vi "Plotter_TDMS.vi"() -> ()   [LabVIEW 2020]
uses:
  General-Controler/panel position.ctl
  Shared/MySQL/Preset Query Enum.ctl
  plotter setup cluster.ctl
  <vilib>/Utility/tcp.llb/UDP Multicast Read-Only Open.vi
  <userlib>/_OpenG.lib/file/file.llb/Convert File Extension (Path)__ogtk.vi
panel:
  in  "Stop button":bool
  in  "Tab Control 2":T1(tab)
  out "parameters to get":string[][](array[string])
  out "devices to get data from":string[](array[string])
  out "Mcast Data":string
  out "scans path":path
  out "TDMS file path":path
  out "Axis Name List":string[](array[string])
  out "All Devices Core Info":string[][](array[string])
  out "UDP Mcast Error":errorcluster
  out "plotter details":string[][](array[string])
  in  "Cluster":T2
  out "appargs":string[](array[string])
  in  "Tab Control":T3(tab)
  out "xy graph":cluster{dbl[], dbl[]}[](graph)
  out "Scan":string
  out "Scan in progress":bool
  out "xy graph bin":cluster{dbl[], dbl[]}[](graph)=[{[5.5, 15.5, 25.5, 35.5, 45.5, 55.5, 0.0], [0.1, 0.1, 0.15, 0.15, 0.2, 0.2, 0.0]}, {[5.5, 5.5, nan, 15.5, 15.5, nan, 25.5, 25.5, nan, 35.5, 35.5, nan, 45.5, 45.5, nan, 55.5, 55.5, nan, 0.0, 0.0, nan], [0.1, 0.1, nan, 0.1, 0.1, nan, 0.15, 0.15, nan, 0.15, 0.15, nan, 0.2, 0.2, nan, 0.2, 0.2, nan, 0.0, 0.0, nan]}, {[5.5, 15.5, 25.5, 35.5, 45.5, 55.5, 0.0], [5.5, 15.5, 25.5, 35.5, 45.5, 55.5, 0.0]}, {[5.5, 5.5, nan, 15.5, 15.5, nan, 25.5, 25.5, nan, 35.5, 35.5, nan, 45.5, 45.5, nan, 55.5, 55.5, nan, 0.0, 0.0, nan], [3.0, 8.0, nan, 13.0, 18.0, nan, 23.0, 28.0, nan, 33.0, 38.0, nan, 43.0, 48.0, nan, 53.0, 58.0, nan, 0.0, 0.0, nan]}]
  in  "Override":bool
  out "Experiment":u16(ring) items=["BaratronProject", "Bella", "ControlRoom", "DataLogging", "Developer", "HeaterTest", "Lanex Bella", "Plasma2", "Test"]
  out "Current State":string
  out "Mcast Path Data":string
  in  "file path":path
  in  "FilePath":bool
  in  "replot":bool
  in  "X Axis":u16(ring)=1
  in  "Y Axis 2":u16(ring)
  in  "Y Axis":u16(ring)
  in  "override":bool
  in  "replot 2":bool
  in  "y axis 2 override":string
  in  "y axis override":string
  in  "x axis override":string
  out "device data Spreadsheet format":string[][](array[string])
  in  "Left":i16=25
  in  "Top":i16=75
  in  "expt_Plotteridfor vi mode":string="46"
  out "Actual expt_plotter.id":string
  out "expt":string
  out "plotter#":string
  out "Screen\nPosition":cluster{"Left":i16, "Top":i16}
  out "x axis name":string
  out "ScanStart ExptName":string
  out "Y Axis Default name":string
  out "MC_IP":string
  out "Path used":path
  out "error out 2":errorcluster
  out "ScanStatus":string
  out "error out 5":errorcluster
  out "s start dat":string
  out "scan end mcast":string
  out "Y Axis Default name 2":string
  out "data":string[][](array[string])
  out "tdms data":string[][](array[string])
  # "17 Fake cam 1 to 5"
  # "15"
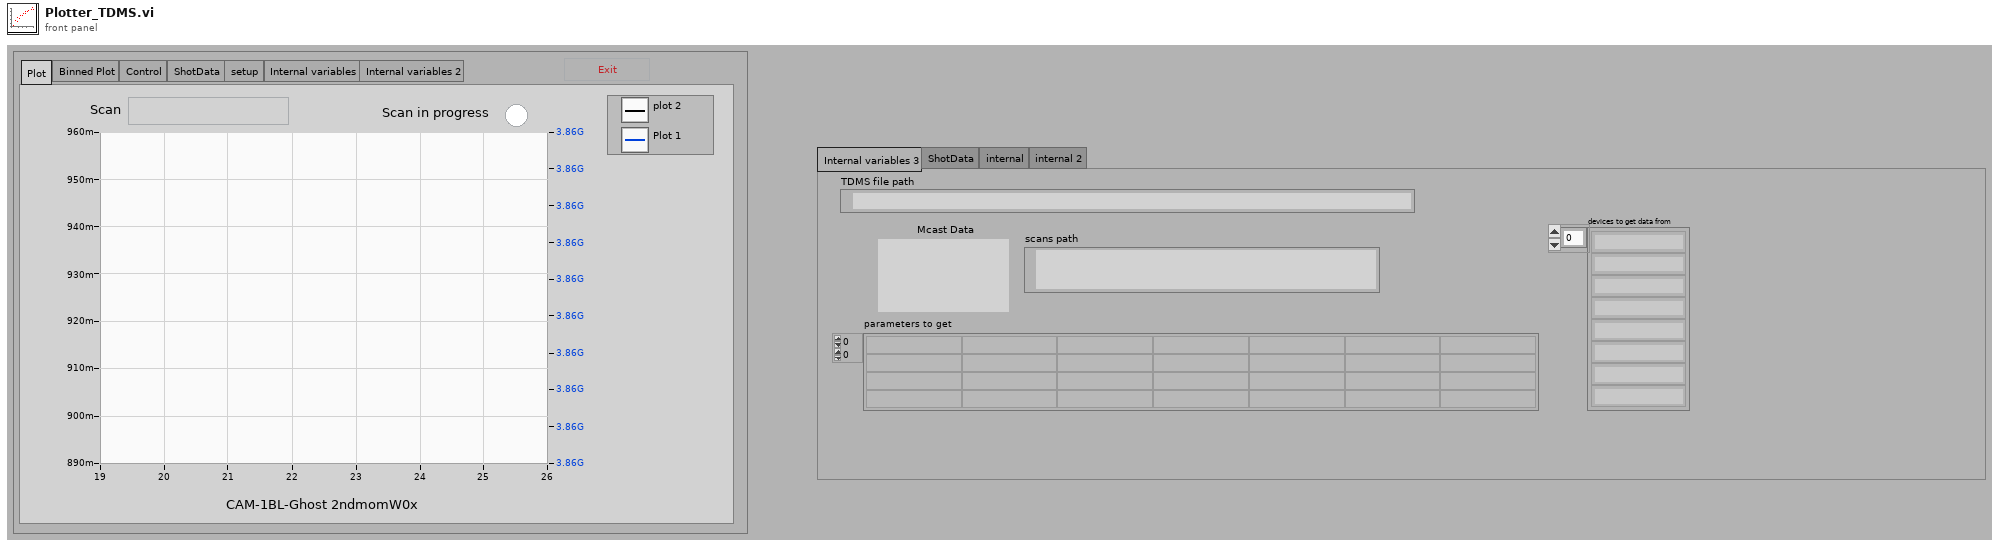
[diagram p1: front panel]
types:
  T1 = enum32{"Internal variables 3", "ShotData", "internal", "internal 2"}
  T2 = typedef "panel position.ctl" = cluster{"Left":i16, "Top":i16, "Width":u32, "Height":u32}
  T3 = enum32{"Plot", "Binned Plot", "Control", "ShotData", "setup", "Internal variables", "Internal variables 2"}
  T4 = typedef "Plotter FGV cluster control.ctl" = cluster{"Multicast Address":string, "Plotter Busy":bool, "Plotter Exit":bool, "Mcast Port":u16}
  T5 = enum32{"invalid app kind", "Development System", "Run Time System", "Student Edition", "Embedded LabVIEW", "Evaluation", "Custom"}
  T6 = enum32{"Invalid", "Standard", "Closed", "Hidden", "Minimized", "Maximized"}
  T7 = typedef "Preset Query Enum.ctl" = enum16{"Get Locations", "Get all IPs and MACs", "Get classes", "Get expt variables to set at scanstart for particular device", "Get expt devices and variables with start values", "Get expt devices and variables (with data to get)", "Get expt devices with data to get", "Get Expt devices and GUIs", "Get all devices basic properties", "Get Virtual Devices Core Info", "Get Expt names", "Get experiment basic properties", "Get experiment alarm variables", "Get MC Ports", "Get device network comm port", "Get devicetype lvclass path", "Get basic device properties", "Get Init Order", "Get all setable variables of a device", "Get device variable aliases", "Get force values of all settable variables", "Get all variables of a devicetype", "Get all variables of a device", "Get plotter details", "Get Saved Scans", "Get Scan Info", "GetGeneralGUIs", "Get expt for plotter", "Get plotter IDs from expt", "Get all devices", "Get all Virtual Devices", "Get all aliases", "Get variable and device info for Virtual Device", "GetItemLocatorIP", "Get IPs for GUIs", "Get DeviceType from Device", "GetLocalPortRange", "GetDevicePresetVariables", "Get Device Configuration", "GetAllPresetNames", "GetAllConfigurationNames", "GetPresetDeviceNames", "GetDeviceAliases", "GetDevicesOfClass"}
  T8 = typedef "plotter setup cluster.ctl" = cluster{"screenx":i16, "screeny":i16, "variable1":string, "variable2":string, "name":string}
  T9 = cluster{"Ring Refnum x":refnum<vi>, "Ring Refnum y":refnum<vi>, "Ring Refnum y 2":refnum<vi>, "XY Graph Refnum":refnum<vi>}
  T10 = cluster{"Core":cluster{"Current VI Reference":refnum<vi>, "Close Panel on Exit?":bool}, "All Devices Core Info":string[][], "Expt Config Files":string[], "Experiment name":string, "ScanData to receive":string[][], "Device Names for scan data":string[], "expt config file array":string[][], "Data titles from config array":string[], "TDMS file path":path, "Plotter setup cluster":T8, "plotter#":string, "bin complete":bool}
  T11 = typedef "LVRectTypeDef.ctl" = cluster{"Left":i16, "Top":i16, "Right":i16, "Bottom":i16}
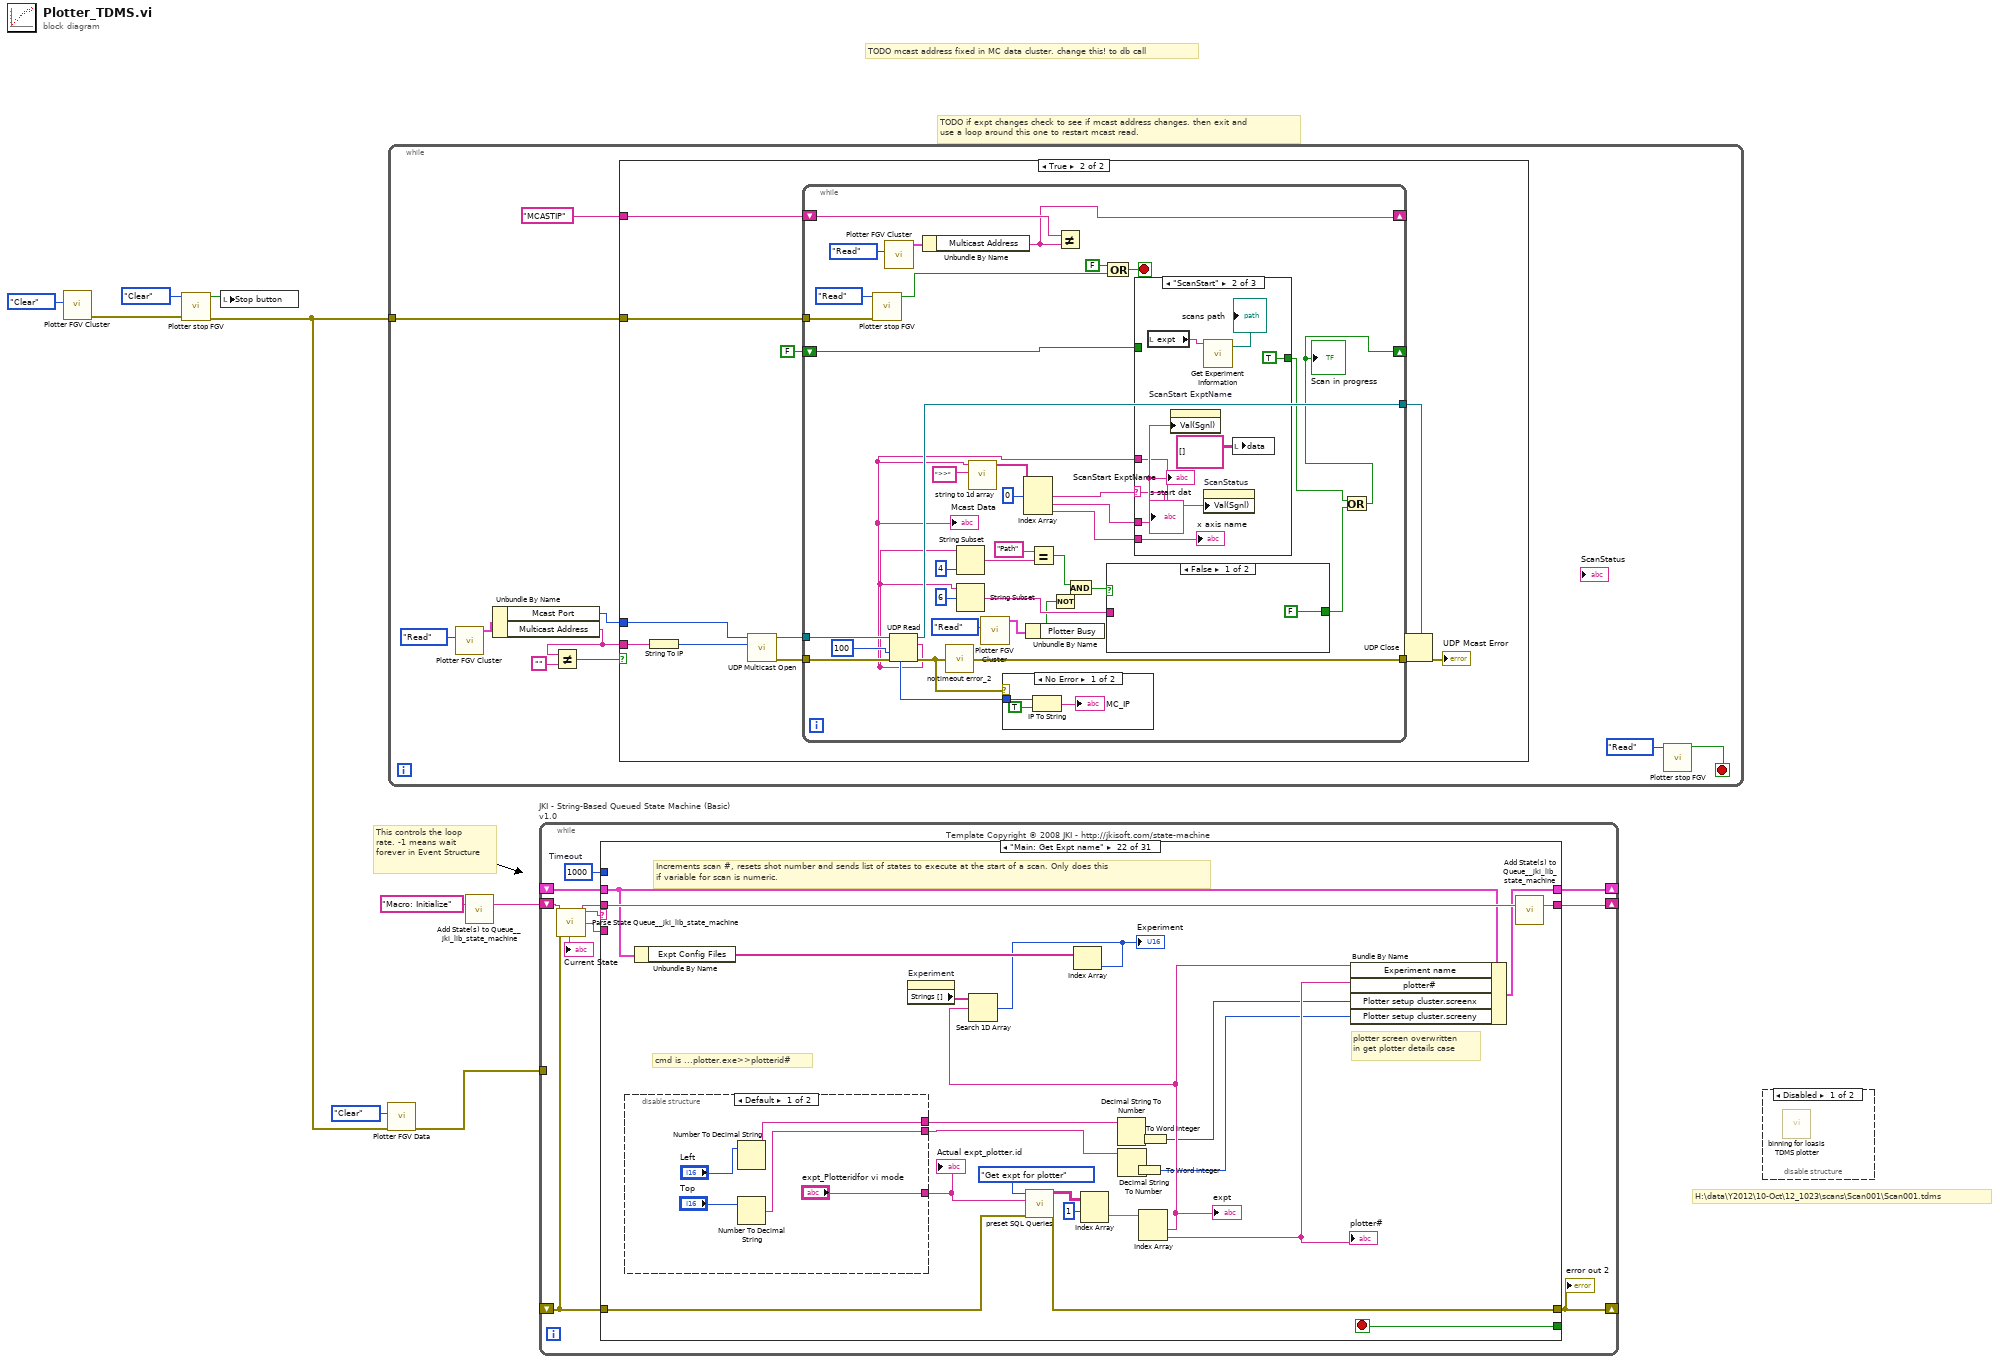
[diagram p0: block diagram]
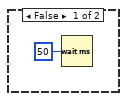
[diagram p3: hidden frame]
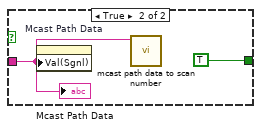
[diagram p5: hidden frame]
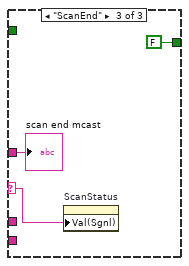
[diagram p7: hidden frame]
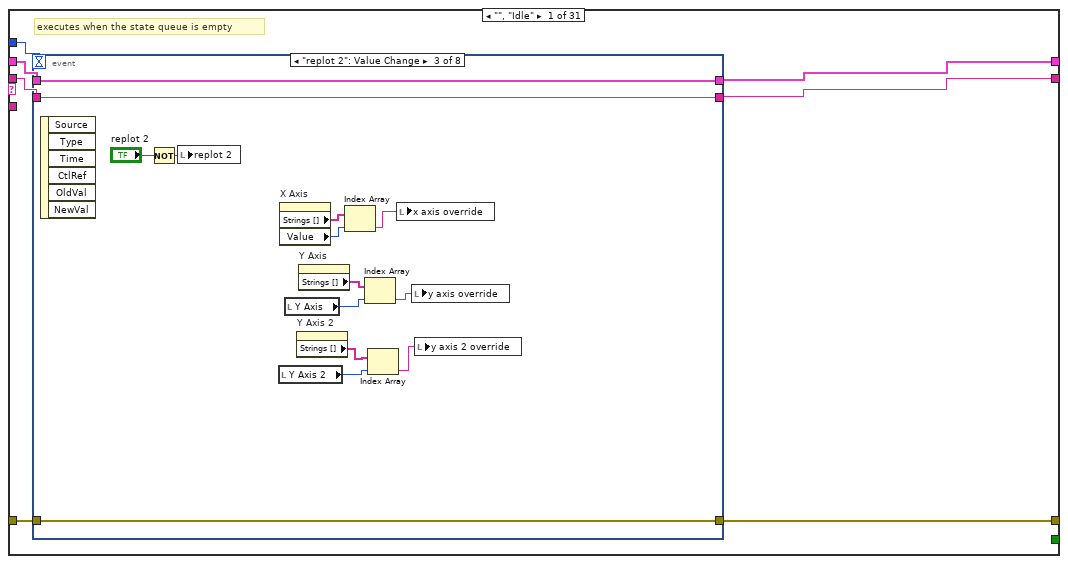
[diagram p8: hidden frame]
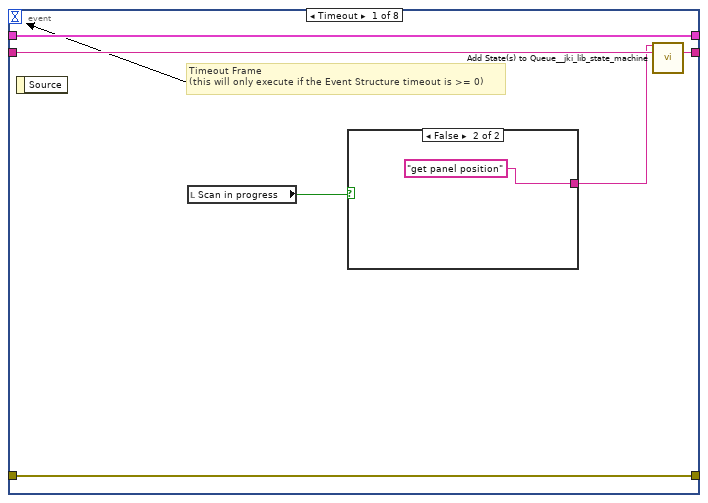
[diagram p9: hidden frame]
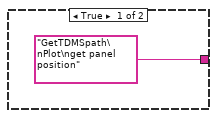
[diagram p10: hidden frame]
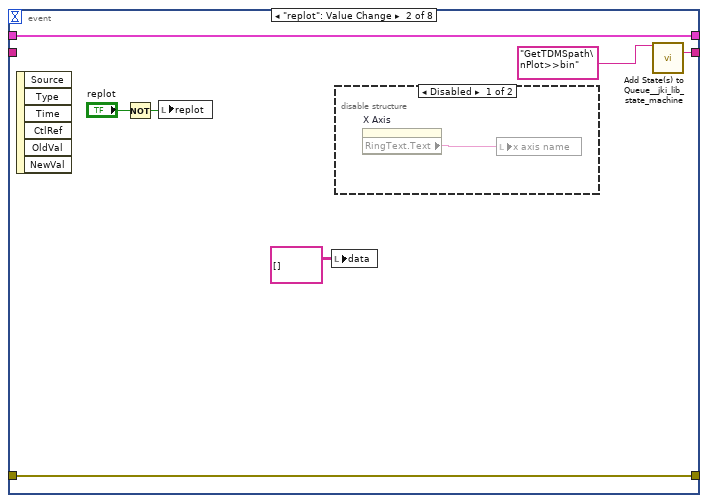
[diagram p11: hidden frame]
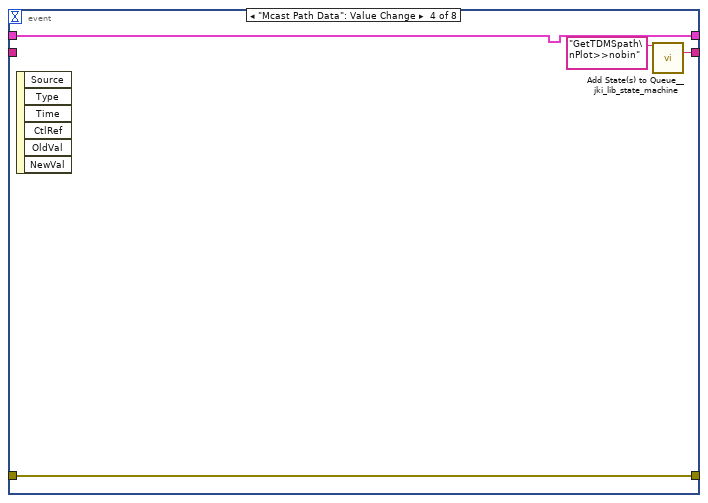
[diagram p13: hidden frame]
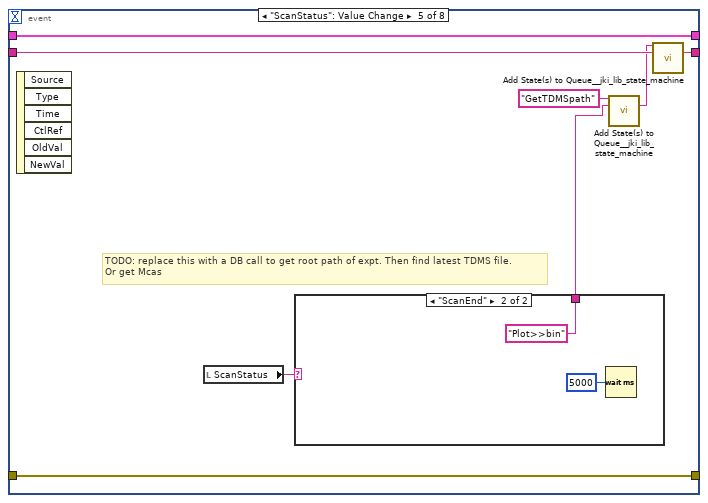
[diagram p14: hidden frame]
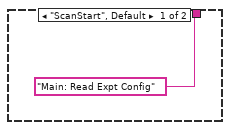
[diagram p15: hidden frame]
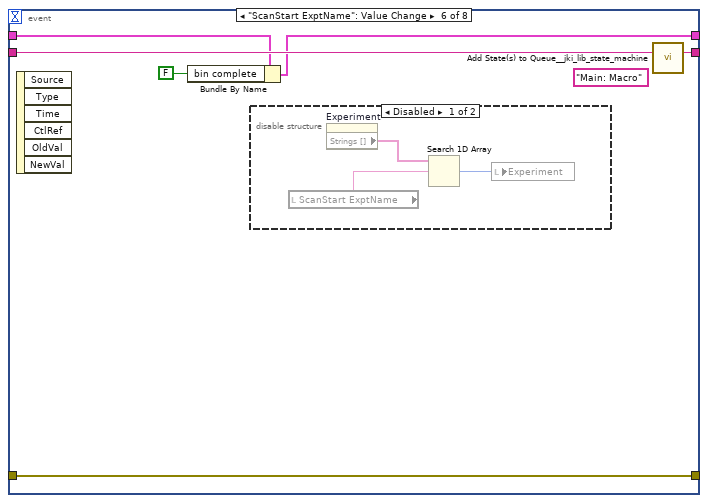
[diagram p16: hidden frame]
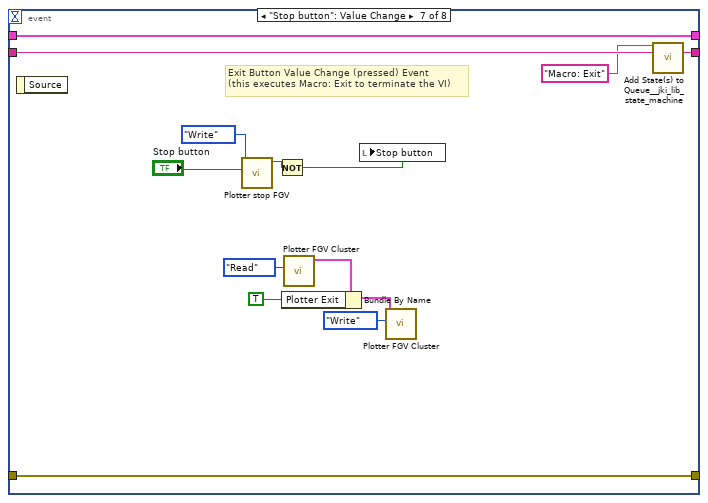
[diagram p18: hidden frame]
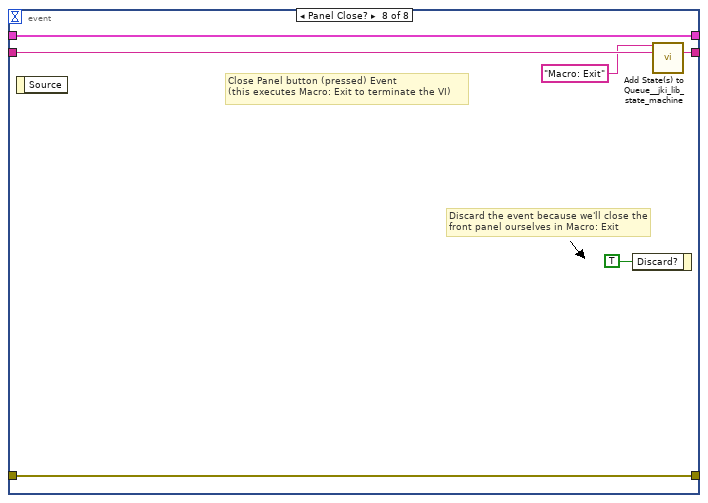
[diagram p19: hidden frame]
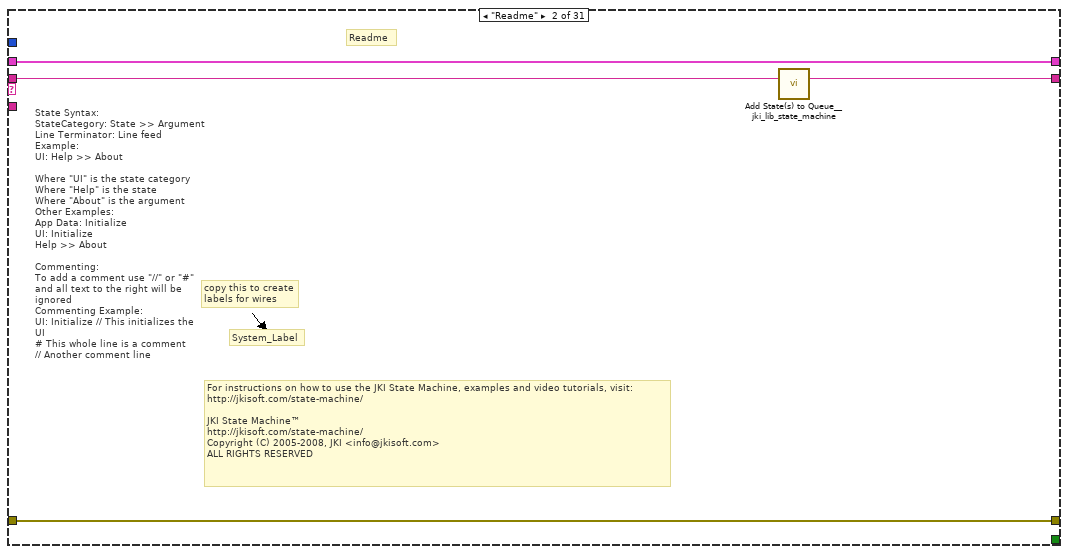
[diagram p20: hidden frame]
diagram:
  # "H:\\data\\Y2012\\10-Oct\\12_1023\\scans\\Scan001\\Scan001.tdms"
  # "TODO mcast address fixed in MC data cluster. change this! to db call"
  # "TODO if expt changes check to see if mcast address changes. then exit and\nuse a loop around this one to restart mcast read."
  # "This controls the loop rate. -1 means wait forever in Event Structure"
  n1 = call "Plotter FGV Cluster.vi"("Function"=enum16{"Read", "Write", "Clear"}."Clear") -> ("error out"=w5:errorcluster)  [unwired: 9 in, 1 out]
  n2 = call "Plotter stop FGV.vi"("error in"=w5, "Function"=enum16{"Read", "Write", "Clear"}."Clear") -> ("error out"=w2:errorcluster, "Stop out"=w4:bool)  [unwired: 8 in]
  n3 = local write "Stop button"(w4) -> ()
  n4 = call "Plotter FGV Data.vi"("error in"=w2, "Function"=enum16{"Read", "Write", "Clear"}."Clear") -> ("error out"=w1:errorcluster)  [unwired: 8 in, 1 out]
  n5 = while {
    tunnel: w2 -> [w13]
    stop <- w17 stop-if-true
    n6 = call "Plotter FGV Cluster.vi"("Function"=enum16{"Read", "Write", "Clear"}."Read") -> ("Cluster out"=w14:T4)  [unwired: 9 in, 1 out]
    n7 = Unbundle By Name(w14) -> ("Mcast Port"=w10:u16, "Multicast Address"=w12:string)
    n8 = Not Equal?(x=w12, y="") -> (x != y?=w16:bool)
    n9 = case shown="True" w16 {
      tunnel: "MCASTIP" ("Multicast Address") -> [_ w25]
      tunnel: w12 -> [_ w24]
      tunnel: w13 -> [_ w23]
      tunnel: w10 -> [_ w22]
      frame False {
        n10 = Wait (ms)(milliseconds to wait=u32 50) -> ()  [unwired: 1 out]
      }
      frame True {
        n11 = String To IP(1:w24) -> (0:w31:u32)
        n12 = call-poly <vilib>:"UDP Multicast Open.vi"("multicast addr"=w31, "port"=w22) -> ("error out"=w26:errorcluster, "connection ID"=w30:refnum<k16>)  [unwired: 7 in, 1 out]
        n13 = while {
          tunnel: w30 -> [w68]
          tunnel: [w67] -> w29
          tunnel: [w66] -> w28
          tunnel: w26 -> [w62]
          tunnel: w23 -> [w60]
          shift-right: [w38] -> _
          shift-left: w25 -> [w49]
          shift-right: [w34] -> _
          shift-left: FALSE -> [w33]
          stop <- w50 stop-if-true
          n14 = call "Plotter stop FGV.vi"("error in"=w60, "Function"=enum16{"Read", "Write", "Clear"}."Read") -> ("Stop out"=w51:bool)  [unwired: 8 in, 1 out]
          n15 = call "Plotter FGV Cluster.vi"("Function"=enum16{"Read", "Write", "Clear"}."Read") -> ("Cluster out"=w48:T4)  [unwired: 9 in, 1 out]
          n16 = UDP Read(connection ID=w68, timeout ms (25000)=100, 8:w62) -> (data out=w37:string, error out=w39:errorcluster, 3:w67:refnum<k16>, 6:w40:u32)  [unwired: 2 out]
          "Mcast Data" <- w37
          n17 = Unbundle By Name(w48) -> ("Multicast Address"=w38:string)
          n18 = call "no timeout error_2.vi"("error in (no error)"=w39) -> ("error out"=w66:errorcluster)
          n19 = String Subset(string=w37, length (rest)=4 ("length (rest)")) -> (substring=w57:string)  [unwired: 1 in]
          n20 = String Subset(string=w37, offset (0)=6) -> (substring=w55:string)  [unwired: 1 in]
          n21 = call "string to 1d array.vi"("delimiter (Tab)"=">>", "string"=w37) -> ("Array of Strings"=w64:string[])  [unwired: 9 in]
          n22 = call "Plotter FGV Cluster.vi"("Function"=enum16{"Read", "Write", "Clear"}."Read") -> ("Cluster out"=w43:T4)  [unwired: 9 in, 1 out]
          n23 = case shown="No Error" w39 {
            tunnel: w40 -> [w72 _]
            frame No Error {
              n24 = IP To String(1:TRUE ("dot notation? (F)"), 2:w72) -> (0:→"MC_IP":string)
            }
            frame Error {
            }
          }
          n25 = Index Array(array=w64, index #1=0 ("index")) -> (element #1=w46:string, element #2=w52:string, element #3=w53:string)  [unwired: 2 in]
          n26 = Unbundle By Name(w43) -> ("Plotter Busy"=w42:bool)
          n27 = Equal?(x="Path" ("y"), y=w57) -> (x = y?=w54:bool)
          n28 = Not(x=w42) -> (.not. x?=w41:bool)
          n29 = Not Equal?(x=w49, y=w38) -> ()  [unwired: 1 out]
          n30 = And(x=w54, y=w41) -> (x .and. y?=w45:bool)
          n31 = case shown="False" w45 {
            tunnel: w55 -> [_ w75]
            tunnel: [FALSE ("Scan in progress") TRUE ("Scan in progress")] -> w35
            frame False {
            }
            frame True {
              n32 = property on="Mcast Path Data" class="Str"("Val(Sgnl)"=w75) -> ()  [unwired: 2 in, 2 out]
              n33 = call "mcast path data to scan number.vi"("mcast path data"=w75) -> ()  [unwired: 10 in, 1 out]
              "Mcast Path Data" <- w75
            }
          }
          n34 = Compound Arithmetic op=OR(FALSE ("value"), w51) -> (w50:bool)
          n35 = case shown="\"ScanStart\"" w46 {
            selector: w46 -> [_ w82 w87]
            tunnel: w53 -> [_ w84 _]
            tunnel: w52 -> [_ w83 _]
            tunnel: w37 -> [_ w81 w86]
            tunnel: [w76 TRUE ("Scan in progress") FALSE ("Scan in progress")] -> w36
            tunnel: w33 -> [w76 _ _]
            frame Default {
            }
            frame "ScanStart" {
              n36 = local read "expt"() -> (w80:string)
              n37 = property on="ScanStart ExptName" class="Str"("Val(Sgnl)"=w83) -> ()  [unwired: 2 in, 2 out]
              n38 = call "Get Experiment Information.vi"("> Expt Name >"=w80) -> ("scans path"=→"scans path":path)  [unwired: 2 in, 8 out]
              n39 = property on="ScanStatus" class="Str"("Val(Sgnl)"=w82) -> ()  [unwired: 2 in, 2 out]
              n40 = local write "data"(string[][] [] ("data")) -> ()
              "x axis name" <- w84
              "ScanStart ExptName" <- w83
              "s start dat" <- w81
            }
            frame "ScanEnd" {
              n41 = property on="ScanStatus" class="Str"("Val(Sgnl)"=w87) -> ()  [unwired: 2 in, 2 out]
              "scan end mcast" <- w86
            }
          }
          n42 = Or(x=w36, y=w35) -> (x .or. y?=w34:bool)
          "Scan in progress" <- w34
        }
        n43 = UDP Close(connection ID=w29, 8:w28) -> (error out=→"UDP Mcast Error":errorcluster)  [unwired: 1 out]
      }
    }
    n44 = call "Plotter stop FGV.vi"("Function"=enum16{"Read", "Write", "Clear"}."Read") -> ("Stop out"=w17:bool)  [unwired: 9 in, 1 out]
  }
  n45 = call <vilib>:"Add State(s) to Queue__jki_lib_state_machine.vi"("State(s) in (\"\")"="Macro: Initialize") -> ("States Out"=w9:string)  [unwired: 14 in]
  n46 = while "JKI - String-Based Queued State Machine (Basic) v1.0" {
    shift-right: [w92] -> _
    shift-left: _ -> [w91]
    shift-right: [w88] -> _
    shift-left: _ -> [w89]
    shift-right: [w94] -> _
    shift-left: w9 -> [w95]
    tunnel: w1 -> [_]
    stop <- w93 stop-if-true
    w90 = 1000  # Timeout
    # "Template Copyright © 2008 JKI - http://jkisoft.com/state-machine"
    n47 = call <vilib>:"Parse State Queue__jki_lib_state_machine.vi"("State Queue"=w95, "Error In (no error)"=w89) -> ("Remaining States"=w97:string, "Current State"=w98:string, "Arguments"=w96:string)  [unwired: 11 in]
    "Current State" <- w98
    n48 = case shown="\"Main: Get Expt name\"" w98 {
      selector: w98 -> [_ _ _ w188 _ _ _ _ _ _ _ _ _ _ _ _ _ _ _ _ _ _ _ _ _ _ _ _ _ _ _]
      tunnel: w97 -> [w105 w183 w187 w192 w210 w217 w222 w226 w230 w236 w240 w244 w250 w261 w287 w292 w298 w318 w322 w327 w338 w360 w393 w422 w435 w450 w472 w514 w541 w657 w667]
      tunnel: w96 -> [_ _ _ _ _ _ _ _ _ _ _ _ w245 w255 _ _ _ _ _ _ _ _ _ _ _ _ _ _ w520 _ _]
      tunnel: w91 -> [w103 w180 w184 w190 w201 w214 w220 w223 _ w231 w237 w242 w248 w257 w284 w288 w294 w316 w319 w324 w335 w358 w379 w420 w428 w447 w470 w511 w539 w654 w665]
      tunnel: [w102 w181 w185 w194 w207 errorcluster {"status"=FALSE, "code"=0, "source"=""} ("error out") w219 w224 w228 w232 w238 w241 w246 w258 w285 w290 w296 w309 w320 w325 w330 w346 w375 w411 w433 w448 w468 w507 w521 w655 w662] -> w88
      tunnel: w89 -> [w101 w181 w185 w193 w207 w211 w219 w224 w228 w233 w238 w241 w247 w259 w285 w290 w296 w309 w320 w325 w331 w347 w376 w401 w433 w448 w469 w508 w522 w655 w663]
      tunnel: [w104 w182 w186 w191 w209 w216 w221 w225 w229 w235 w239 w243 w249 w260 w286 w291 w297 w317 w321 w326 w337 w359 w392 w421 w434 w449 w471 w513 w540 w656 w666] -> w94
      tunnel: [_ _ _ _ _ _ TRUE _ _ _ _ _ _ _ _ _ _ _ _ _ _ _ _ _ _ _ _ _ _ _ _] -> w93
      tunnel: [w100 w180 w184 w190 w208 w214 w220 w223 w227 w231 w237 w242 w248 w257 w284 w288 w293 w316 w319 w324 w334 w357 w378 w419 w427 w447 w470 w512 w539 w654 w665] -> w92
      tunnel: w90 -> [w99 _ _ _ _ _ _ _ _ _ _ _ _ _ _ _ _ _ _ _ _ _ _ _ _ _ _ _ _ _ _]
      frame "", "Idle" {
        # "executes when the state queue is empty"
        n49 = event shown="[2] \"replot 2\": Value Change" {
          selector: _ -> [_ _ _ _ _ _ _ _]
          dyn-events: _ -> [_ _ _ _ _ _ _ _]
          timeout: w99 -> [_ _ _ _ _ _ _ _]
          tunnel: w105 -> [w111 _ w131 _ w145 w156 w173 w179]
          tunnel: [w110 w120 w131 w139 w147 w155 w172 w178] -> w104
          tunnel: w103 -> [w108 w115 w132 w136 w142 w152 w170 w176]
          tunnel: [w109 w119 w135 w138 w146 w154 w171 w177] -> w102
          tunnel: w101 -> [w109 w119 w135 w138 w146 w154 w171 w177]
          tunnel: [w108 w115 w132 w136 w142 w151 w170 w176] -> w100
          event Timeout {
            # "Timeout Frame\n(this will only execute if the Event Structure timeout is >= 0)"
            n50 = event-data() -> ()  [unwired: 1 in, 1 out]
            n51 = local read "Scan in progress"() -> (w106:bool)
            n52 = case shown="False" w106 {
              tunnel: ["GetTDMSpath\nPlot\nget panel position" "get panel position"] -> w107
              frame True {
              }
              frame False {
              }
            }
            n53 = call <vilib>:"Add State(s) to Queue__jki_lib_state_machine.vi"("State(s) in Front (\"\")"=w107, "State(s) in (\"\")"=w111) -> ("States Out"=w110:string)  [unwired: 13 in]
          }
          event "replot": Value Change {
            n54 = event-data() -> ()  [unwired: 1 in, 6 out]
            n55 = Not(x="replot") -> (.not. x?=w116:bool)
            n56 = local write "replot"(w116) -> ()
            n57 = local write "data"(string[][] [] ("data")) -> ()
            n58 = disable-structure shown="Disabled" {
              frame Disabled {
                n59 = property on="X Axis" class="Ring (strict)"() -> ("RingText.Text"=w121:string)  [unwired: 2 in, 2 out]
                n60 = local write "x axis name"(w121) -> ()
              }
              frame Enabled {
              }
            }
            n61 = call <vilib>:"Add State(s) to Queue__jki_lib_state_machine.vi"("State(s) in Front (\"\")"="GetTDMSpath\nPlot>>bin" ("State(s) in Front (\"\")")) -> ("States Out"=w120:string)  [unwired: 14 in]
          }
          event "replot 2": Value Change {
            n62 = event-data() -> ()  [unwired: 1 in, 6 out]
            n63 = Not(x="replot 2") -> (.not. x?=w133:bool)
            n64 = local write "replot 2"(w133) -> ()
            n65 = local read "Y Axis 2"() -> (w125:u16)
            n66 = property on="X Axis" class="Ring (strict)"() -> ("Strings []"=w128:string[], "Value"=w129:u16)  [unwired: 2 in, 2 out]
            n67 = local read "Y Axis"() -> (w123:u16)
            n68 = property on="Y Axis 2" class="Ring (strict)"() -> ("Strings []"=w124:string[])  [unwired: 2 in, 2 out]
            n69 = property on="Y Axis" class="Ring (strict)"() -> ("Strings []"=w122:string[])  [unwired: 2 in, 2 out]
            n70 = Index Array(array=w128, index=w129) -> (element=w130:string)
            n71 = Index Array(array=w122, index=w123) -> (element=w126:string)
            n72 = Index Array(array=w124, index=w125) -> (element=w127:string)
            n73 = local write "x axis override"(w130) -> ()
            n74 = local write "y axis override"(w126) -> ()
            n75 = local write "y axis 2 override"(w127) -> ()
          }
          event "Mcast Path Data": Value Change {
            n76 = event-data() -> ()  [unwired: 1 in, 6 out]
            n77 = call <vilib>:"Add State(s) to Queue__jki_lib_state_machine.vi"("State(s) in Front (\"\")"="GetTDMSpath\nPlot>>nobin" ("State(s) in Front (\"\")")) -> ("States Out"=w139:string)  [unwired: 14 in]
          }
          event "ScanStatus": Value Change {
            # "TODO: replace this with a DB call to get root path of expt. Then find latest TDMS file.\nOr get Mcas"
            n78 = event-data() -> ()  [unwired: 1 in, 6 out]
            n79 = local read "ScanStatus"() -> (w144:string)
            n80 = case shown="\"ScanEnd\"" w144 {
              tunnel: ["Main: Read Expt Config" ("State(s) in Front (\"\")") "Plot>>bin" ("State(s) in Front (\"\")")] -> w141
              frame "ScanStart", Default {
              }
              frame "ScanEnd" {
                n81 = Wait (ms)(milliseconds to wait=u32 5000) -> ()  [unwired: 1 out]
              }
            }
            n82 = call <vilib>:"Add State(s) to Queue__jki_lib_state_machine.vi"("State(s) in Front (\"\")"="GetTDMSpath" ("State(s) in Front (\"\")"), "State(s) in (\"\")"=w141) -> ("States Out"=w140:string)  [unwired: 13 in]
            n83 = call <vilib>:"Add State(s) to Queue__jki_lib_state_machine.vi"("State(s) in Front (\"\")"=w140, "State(s) in (\"\")"=w145) -> ("States Out"=w147:string)  [unwired: 13 in]
          }
          event "ScanStart ExptName": Value Change {
            (unwired) "Main: Macro"
            n84 = event-data() -> ()  [unwired: 1 in, 6 out]
            n85 = Bundle By Name(cluster=w152, "bin complete"=FALSE) -> (w151:T10)
            n86 = disable-structure shown="Disabled" {
              frame Disabled {
                n87 = local read "ScanStart ExptName"() -> (w158:string)
                n88 = property on="Experiment" class="Ring (strict)"() -> ("Strings []"=w159:string[])  [unwired: 2 in, 2 out]
                n89 = Search 1D Array(1D array=w159, element=w158) -> (index of element=w157:i32)  [unwired: 1 in]
                n90 = local write "Experiment"(w157) -> ()
              }
              frame Enabled {
              }
            }
            n91 = call <vilib>:"Add State(s) to Queue__jki_lib_state_machine.vi"("State(s) in (\"\")"=w156) -> ("States Out"=w155:string)  [unwired: 14 in]
          }
          event "Stop button": Value Change {
            # "Exit Button Value Change (pressed) Event\n(this executes Macro: Exit to terminate the VI)"
            n92 = event-data() -> ()  [unwired: 1 in, 1 out]
            n93 = call "Plotter stop FGV.vi"("Stop in"="Stop button", "Function"=enum16{"Read", "Write", "Clear"}."Write") -> ("Stop out"=w167:bool)  [unwired: 8 in, 1 out]
            n94 = Not(x=w167) -> (.not. x?=w166:bool)
            n95 = call "Plotter FGV Cluster.vi"("Function"=enum16{"Read", "Write", "Clear"}."Read") -> ("Cluster out"=w162:T4)  [unwired: 9 in, 1 out]
            n96 = Bundle By Name(cluster=w162, "Plotter Exit"=TRUE) -> (w160:T4)
            n97 = local write "Stop button"(w166) -> ()
            n98 = call "Plotter FGV Cluster.vi"("Function"=enum16{"Read", "Write", "Clear"}."Write", "Cluster in"=w160) -> ()  [unwired: 8 in, 2 out]
            n99 = call <vilib>:"Add State(s) to Queue__jki_lib_state_machine.vi"("State(s) in Front (\"\")"="Macro: Exit", "State(s) in (\"\")"=w173) -> ("States Out"=w172:string)  [unwired: 13 in]
          }
          event Panel Close? {
            # "Discard the event because we'll close the front panel ourselves in Macro: Exit"
            # "Close Panel button (pressed) Event\n(this executes Macro: Exit to terminate the VI)"
            n100 = event-data() -> ()  [unwired: 1 in, 1 out]
            n101 = event-data("Discard?"=TRUE) -> ()  [unwired: 1 in, 1 out]
            n102 = call <vilib>:"Add State(s) to Queue__jki_lib_state_machine.vi"("State(s) in Front (\"\")"="Macro: Exit", "State(s) in (\"\")"=w179) -> ("States Out"=w178:string)  [unwired: 13 in]
          }
        }
      }
      frame "Readme" {
        # "For instructions on how to use the JKI State Machine, examples and video tutorials, visit:\nhttp://jkisoft.com/state-machine/\n\nJKI State Machine™\nhttp://jkisoft.com/state-machine/\nCopyright (C) 2005-2008, JKI <info@jkisoft.com>\nALL RIGHTS RESERVED"
        # "copy this to create labels for wires"
        # "System_Label"
        # "State Syntax:\nStateCategory: State >> Argument\nLine Terminator: Line feed\nExample:\nUI: Help >> About\n\nWhere \"UI\" is the state category\nWhere \"Help\" is the state\nWhere \"About\" is the argument\nOther Examples:\nApp Data: Initialize\nUI: Initialize\nHelp >> About\n\nCommenting:\nTo add a comment use \"//\" or \"#\" and all text to the right will be ignored\nCommenting Example:\nUI: Initialize // This initializes the UI\n# This whole line is a comment\n// Another comment line"
        # "Readme"
        n103 = call <vilib>:"Add State(s) to Queue__jki_lib_state_machine.vi"("State(s) in (\"\")"=w183) -> ("States Out"=w182:string)  [unwired: 14 in]
      }
      frame "---------- Core ----------" {
        # "Do not put any code in this frame.\n(it is a separator no-op)"
        n104 = call <vilib>:"Add State(s) to Queue__jki_lib_state_machine.vi"("State(s) in (\"\")"=w187) -> ("States Out"=w186:string)  [unwired: 14 in]
      }
      frame Default {
        w197 = 42 items=["No error", "Argument error", "Memory is full", "Out of zone", "End of file", "File already open", "Generic file I/O error", "File not found", "File permission error", "Disk is full", "Duplicate path", "Too many files open", "System feature not enabled", "Resource file not found", "Cannot add resource", "Resource not found", "Image not found", "Image memory error", "Pen does not exist", "Config type invalid", "Config token not found", "Config parse error", "Config memory error", "Bad external code format", "Bad external code offset", "External code not present", "Null window", "Destroy window error", "Null menu", "Print aborted", "Bad print record", "Print driver error", "Windows error during printing", "Memory error during printing", "Print dialog error", "Generic print error", "Invalid device refnum", "Device not found", "Device parameter error", "Device unit error", "Cannot open device", "Device call aborted", "Generic error", "Cancelled by user", "Object ID too low", "Object ID too high", "Object not in heap", "Unknown heap", "Unknown object (invalid DefProc)", "Unknown object (DefProc not in table)", "Message out of range", "Invalid (null) method", "Unknown message", "Manager call not supported", "Bad address", "Network operation in progress", "Network operation timed out", "Connection is busy", "Network attribute not supported", "Network error", "Address in use", "System out of memory", "Connection aborted", "Connection refused", "Not connected", "Already connected", "Connection closed", "Initialization error (interapplication manager)", "Bad occurrence", "Wait on unbound occurrence handler", "Occurrence queue overflow", "Datalog type conflict", "Unused", "Unrecognized type (interapplication manager)", "Memory corrupt", "Failed to make temporary DLL", "Old CIN version", "Drag socket not found", "Failed to load drop-object", "Failed to register OLE object", "Failed to release OLE object", "Format specifier type mismatch", "Unknown format specifier", "Too few format specifiers", "Too many format specifiers", "Scan failed", "Newer CIN version", "Error converting to variant", "Runtime menu error", "Password tampered", "Variant attribute not found", "Incompatible variant data type", "Event data is not available", "Event Store is not present", "Occurrence is not found", "Event Queue is not created", "Event info is not available", "Refnum passed is NULL", "Error retrieving Class GUID", "Error retrieving CoClass GUID", "Error retrieving TypeLib GUID.", "Bad built application magic bytes.", "Specific driver is different from the specific driver associated with the Logical Name.", "There is no session opened to the class driver.", "Max Error", "MAX - Error with config objects", "MAX - Error loading configuration", "MAX - Group not supported"]
        # "Current State"
        # "Do not delete, rename, or modify this frame.\n(this is used to capture unhandled states and typos)"
        # "Handle mistyped state name (developer tool)"
        n105 = Format Into String(format string="Software Exception: Unhandled State \"%s\"." ("message"), error in=w193, w188) -> (resulting string=w196:string, error out=w195:errorcluster)  [unwired: 1 in]
        n106 = call <vilib>:"Error Cluster From Error Code.vi"("show call chain? (False)"=TRUE, "error in (no error)"=w195, "error message (\"\")"=w196, "error code (0)"=w197) -> ("error out"=w194:errorcluster)  [unwired: 5 in]
        n107 = call <vilib>:"Add State(s) to Queue__jki_lib_state_machine.vi"("State(s) in (\"\")"=w192) -> ("States Out"=w191:string)  [unwired: 14 in]
      }
      frame "Initialize Core Data" {
        # "Do not delete, rename, or modify this frame.\n(this is used to determine panel behavior on exit)"
        # "originally closed?"
        # "exe?"
        # "If panel starts closed or is an EXE, then close it when we exit"
        n108 = property class="VI"() -> ("Front Panel.Open"=w206:bool)  [unwired: 2 in, 2 out]
        n109 = property class="App"() -> ("App.Kind"=w205:T5)  [unwired: 2 in, 2 out]
        n110 = control-ref of="Current VI Reference"() -> (w199:refnum<vi>)
        n111 = Not(x=w206) -> (.not. x?=w203:bool)
        n112 = Equal?(x=w205, y=T5."Run Time System" ("Application:Kind")) -> (x = y?=w202:bool)
        n113 = Or(x=w203, y=w202) -> (x .or. y?=w200:bool)
        n114 = Bundle By Name(cluster=w201, "Core.Current VI Reference"=w199, "Core.Close Panel on Exit?"=w200) -> (w208:T10)
        n115 = call <vilib>:"Add State(s) to Queue__jki_lib_state_machine.vi"("State(s) in (\"\")"=w210) -> ("States Out"=w209:string)  [unwired: 14 in]
      }
      frame "Error Handler" {
        # "Unhandled Error -- Display it"
        # "Handle any errors here.\nYou can also output any states to clean-up after errors occur"
        # "Clear error"
        n116 = Wait (ms)(milliseconds to wait=u32 1500) -> ()  [unwired: 1 out]
        n117 = call <vilib>:"Add State(s) to Queue__jki_lib_state_machine.vi"("State(s) in Front (\"\")"="/* Post Error States", "State(s) in (\"\")"=w217) -> ("States Out"=w216:string)  [unwired: 13 in]
        "error out 5" <- w211
      }
      frame "Exit" {
        # "Do not put any code in this frame.\n(No errors that occur here will be handled.)"
        n118 = call <vilib>:"Add State(s) to Queue__jki_lib_state_machine.vi"("State(s) in (\"\")"=w222) -> ("States Out"=w221:string)  [unwired: 14 in]
      }
      frame "---------- Data ----------" {
        # "Do not put any code in this frame.\n(It is a separator no-op. You can make a copy of this frame to create a new Data frame)"
        n119 = call <vilib>:"Add State(s) to Queue__jki_lib_state_machine.vi"("State(s) in (\"\")"=w226) -> ("States Out"=w225:string)  [unwired: 14 in]
      }
      frame "Data: Initialize" {
        # "Initialize the shift-register data, here.\n(data names are defined by what you wire into the bundle function)"
        n120 = call "Data Cluster Plotter.vi"() -> ("output cluster"=w227:T10)
        n121 = call <vilib>:"Add State(s) to Queue__jki_lib_state_machine.vi"("State(s) in (\"\")"=w230) -> ("States Out"=w229:string)  [unwired: 14 in]
      }
      frame "Data: Cleanup" {
        # "Cleanup any data and references, here.\n(this is called automatically, by the Macro: Exit)"
        n122 = Unbundle By Name(w231) -> ("Core.Current VI Reference"=w234:refnum<vi>)
        n123 = Close Reference(reference=w234, error in (no error)=w233) -> (error out=w232:errorcluster)
        n124 = call <vilib>:"Add State(s) to Queue__jki_lib_state_machine.vi"("State(s) in (\"\")"=w236) -> ("States Out"=w235:string)  [unwired: 14 in]
      }
      frame "---------- UI ----------" {
        # "Do not put any code in this frame.\n(It is a separator no-op. You can make a copy of this frame to create a new UI frame)"
        n125 = call <vilib>:"Add State(s) to Queue__jki_lib_state_machine.vi"("State(s) in (\"\")"=w240) -> ("States Out"=w239:string)  [unwired: 14 in]
      }
      frame "UI: Initialize" {
        # "Initialize the User Interface, here.\n(this is called automatically, by the Macro: Init)"
        n126 = call <userlib>:"Fit VI window to Largest Dec__ogtk.vi"() -> ()  [unwired: 6 in, 2 out]
        n127 = call <vilib>:"Add State(s) to Queue__jki_lib_state_machine.vi"("State(s) in (\"\")"=w244) -> ("States Out"=w243:string)  [unwired: 14 in]
      }
      frame "UI: Cursor Set" {
        # "Argument"
        # "Set and Unset Cursor Busy.\n(Usage: \"UI: Cursor Set >> Busy|Idle\")"
        n128 = case shown="\"Idle\", Default" w245 {
          tunnel: w247 -> [w252 w254]
          tunnel: [w251 w253] -> w246
          frame "Idle", Default {
            n129 = call <vilib>:"Unset Busy.vi"("error in (no error)"=w252) -> ("error out"=w251:errorcluster)  [unwired: 10 in]
          }
          frame "Busy" {
            n130 = call <vilib>:"Set Busy.vi"("error in (no error)"=w254) -> ("error out"=w253:errorcluster)  [unwired: 9 in, 1 out]
          }
        }
        n131 = call <vilib>:"Add State(s) to Queue__jki_lib_state_machine.vi"("State(s) in (\"\")"=w250) -> ("States Out"=w249:string)  [unwired: 14 in]
      }
      frame "UI: Front Panel State" {
        # "Argument"
        # "Set Front Panel Open or Closed\n(Usage: \"UI: Front Panel State >> Open|Close\")"
        n132 = Unbundle By Name(w257) -> ("Core.Current VI Reference"=w256:refnum<vi>)
        n133 = case shown="\"Open\", Default" w255 {
          tunnel: w259 -> [w265 w278]
          tunnel: [w267 w279] -> w258
          tunnel: w256 -> [w266 w276]
          frame "Open", Default {
            n134 = property class="VI"(reference=w266, error in=w265) -> (reference out=w263:refnum<vi>, error out=w264:errorcluster, "Front Panel.Open"=w262:bool)
            n135 = case shown="True" w262 {
              tunnel: [w270 w273] -> w267
              tunnel: w264 -> [w269 w273]
              tunnel: w263 -> [w268 _]
              frame False {
                n136 = invoke class="VI" method="FP.Open"(reference=w268, error in=w269, "Activate"=TRUE, "State"=T6."Standard") -> (error out=w270:errorcluster)  [unwired: 1 in, 4 out]
              }
              frame True {
              }
            }
          }
          frame "Close" {
            n137 = property class="VI"(reference=w276, error in=w278) -> (reference out=w275:refnum<vi>, error out=w277:errorcluster, "Front Panel.Open"=w274:bool)
            n138 = case shown="True" w274 {
              tunnel: [w280 w283] -> w279
              tunnel: w277 -> [w280 w282]
              tunnel: w275 -> [_ w281]
              frame False {
              }
              frame True {
                n139 = invoke class="VI" method="FP.Close"(reference=w281, error in=w282) -> (error out=w283:errorcluster)  [unwired: 1 in, 2 out]
              }
            }
          }
        }
        n140 = call <vilib>:"Add State(s) to Queue__jki_lib_state_machine.vi"("State(s) in (\"\")"=w261) -> ("States Out"=w260:string)  [unwired: 14 in]
      }
      frame "---------- Macro ----------" {
        # "Do not put any code in this frame.\n(It is a separator no-op. You can make a copy of this frame to create a new Macro frame)"
        n141 = call <vilib>:"Add State(s) to Queue__jki_lib_state_machine.vi"("State(s) in (\"\")"=w287) -> ("States Out"=w286:string)  [unwired: 14 in]
      }
      frame "Macro: Initialize" {
        w289 = "Data: Initialize\nInitialize Core Data\nUI: Initialize\nUI: Front Panel State >> Open\nMain: Macro"  # Data: Initialize Initialize Core Data UI: Initialize UI: Front Panel State >> Open Main: Macro
        # "Initialization Macro\n(This is called once, when the VI starts)"
        n142 = call <vilib>:"Add State(s) to Queue__jki_lib_state_machine.vi"("State(s) in Front (\"\")"=w289, "State(s) in (\"\")"=w292) -> ("States Out"=w291:string)  [unwired: 13 in]
      }
      frame "GetTDMSpath" {
        # "TODO: replace this with a DB call to get root path of expt. Then find latest TDMS file.\nOr get Mcas"
        n143 = disable-structure shown="Enabled" {
          disable-tunnel: [w306 w307] -> w295
          frame Disabled {
            n144 = local read "MC_IP"() -> (w304:string)
            n145 = local read "Mcast Path Data"() -> (w305:string)
            n146 = Concatenate Strings("\\\\" ("string"), w304) -> (w303:string)
            n147 = Search and Replace String(case sensitive?=TRUE ("ignore case? (F)"), input string=w305, search string="c:" ("string"), replace string=w303) -> (result string=w302:string)  [unwired: 4 in, 3 out]
            n148 = call "MCAST string to TDMS path.vi"("MCAST path"=w302) -> ("TDMS path"=w306:path)  [unwired: 10 in]
          }
          frame Enabled {
            n149 = local read "scans path"() -> (w308:path)
            n150 = call "get latest tdms path.vi"("scans path"=w308) -> ("latest tdms"=w307:path)  [unwired: 10 in]
          }
        }
        n151 = Bundle By Name(cluster=w294, "TDMS file path"=w295) -> (w293:T10)
        n152 = call <vilib>:"Add State(s) to Queue__jki_lib_state_machine.vi"("State(s) in (\"\")"=w298) -> ("States Out"=w297:string)  [unwired: 14 in]
      }
      frame "Macro: Exit" {
        # "Exit Macro\n(This is called once, when the VI exits)"
        n153 = Unbundle By Name(w316) -> ("Core.Close Panel on Exit?"=w315:bool)
        n154 = Select(t="UI: Front Panel State >> Close", s=w315, f="") -> (s? t:f=w312:string)
        n155 = call <vilib>:"Add State(s) to Queue__jki_lib_state_machine.vi"("State(s) in (\"\")"=w312, "State(s) at Back (\"\")"="Data: Cleanup\nExit") -> ("States Out"=w310:string)  [unwired: 13 in]
        n156 = call <vilib>:"Add State(s) to Queue__jki_lib_state_machine.vi"("State(s) in Front (\"\")"=w310, "State(s) in (\"\")"=w318) -> ("States Out"=w317:string)  [unwired: 13 in]
      }
      frame "---------- Main ----------" {
        # "Template Separator\n(You can make a copy of, or modify, this frame)"
        n157 = call <vilib>:"Add State(s) to Queue__jki_lib_state_machine.vi"("State(s) in (\"\")"=w322) -> ("States Out"=w321:string)  [unwired: 14 in]
      }
      frame "Main: Macro" {
        # "Sets the list of states to execute on vi startup in the first string and  the list of states to execute on each loop\nin the second string"
        n158 = flat-sequence {
          frame #0 {
            n159 = local write "Tab Control"(2) -> ()
          }
          frame #1 {
            n160 = local write "Tab Control"(0) -> ()
          }
        }
        n161 = call <vilib>:"Add State(s) to Queue__jki_lib_state_machine.vi"("State(s) in Front (\"\")"="Main: Read Expt Configs\nMain: Get Expt name\nGet plotter details\nMain: Read Expt Config\nGet List of Axis Names\nGet Default Y Axis\nMain: Set Panel Postion\nMain: Get Device Configs", "State(s) in (\"\")"=w327) -> ("States Out"=w326:string)  [unwired: 13 in]
      }
      frame "Main: Read Expt Configs" {
        # "Gets experimental configuration filenames. These files contain information specific to an experiment. Eg TREX expt\nfile would have all the devices that need to startup and their default variable values."
        n162 = call "preset SQL Queries.vi"("error in (no error)"=w331, "Preset Query"=Preset_Query_Enum."Get Expt names") -> ("error out"=w330:errorcluster, "1st column 1st data"=w332:string[])  [unwired: 7 in, 1 out]
        n163 = call "array to strings and values for ring.vi"("list of variables"=w332) -> ("Array"=w336:cluster{"String":string, i32}[])
        n164 = property on="Experiment" class="Ring (strict)"("StringsAndValues[]"=w336) -> ()  [unwired: 2 in, 2 out]
        n165 = Bundle By Name(cluster=w335, "Expt Config Files"=w332) -> (w334:T10)
        n166 = call <vilib>:"Add State(s) to Queue__jki_lib_state_machine.vi"("State(s) in (\"\")"=w338) -> ("States Out"=w337:string)  [unwired: 14 in]
      }
      frame "Main: Get Expt name" {
        # "plotter screen overwritten \nin get plotter details case"
        # "cmd is ...plotter.exe>>plotterid#"
        # "Increments scan #, resets shot number and sends list of states to execute at the start of a scan. Only does this\nif variable for scan is numeric."
        n167 = disable-structure shown="Default" {
          disable-tunnel: ["expt_Plotteridfor vi mode" w372] -> w341
          disable-tunnel: [w363 w367] -> w345
          disable-tunnel: [w361 w366] -> w343
          frame condition #0 (active) {
            n168 = Number To Decimal String(number="Left") -> (decimal integer string=w363:string)  [unwired: 1 in]
            n169 = Number To Decimal String(number="Top") -> (decimal integer string=w361:string)  [unwired: 1 in]
          }
          frame condition #1 {
            n170 = control-ref of="This Application"() -> (w373:refnum<vi>)
            n171 = property class="App"(reference=w373) -> ("App.Args"=w371:string[])  [unwired: 1 in, 2 out]
            "appargs" <- w371
            n172 = Index Array(array=w371, index #1=2 ("index"), index #2=3 ("index"), index #3=4 ("index")) -> (element #1=w372:string, element #2=w367:string, element #3=w366:string)
          }
        }
        "Actual expt_plotter.id" <- w341
        n173 = Unbundle By Name(w358) -> ("Expt Config Files"=w356:string[])
        n174 = property on="Experiment" class="Ring (strict)"() -> ("Strings []"=w350:string[])  [unwired: 2 in, 2 out]
        n175 = call "preset SQL Queries.vi"("error in (no error)"=w347, "Device/Devicetype name\n/Plotter.id/ScanName#"=w341, "Preset Query"=Preset_Query_Enum."Get expt for plotter") -> ("error out"=w346:errorcluster, "data"=w353:string[][])  [unwired: 6 in, 1 out]
        n176 = Index Array(array=w353, index (row)=1) -> (element=w355:string[])  [unwired: 1 in]
        n177 = Decimal String To Number(string=w345) -> (number=w344:i32)  [unwired: 2 in, 1 out]
        n178 = Decimal String To Number(string=w343) -> (number=w342:i32)  [unwired: 2 in, 1 out]
        n179 = To Word Integer(number=w342) -> (16bit integer=w339:i16)
        n180 = Index Array(array=w355) -> (element #1=w348:string, element #2=w351:string)  [unwired: 2 in]
        "expt" <- w348
        "plotter#" <- w351
        n181 = Search 1D Array(1D array=w350, element=w348) -> (index of element=w349:i32)  [unwired: 1 in]
        "Experiment" <- w349
        n182 = Index Array(array=w356, index=w349) -> ()  [unwired: 1 out]
        n183 = To Word Integer(number=w344) -> (16bit integer=w340:i16)
        n184 = Bundle By Name(cluster=w358, "Experiment name"=w348, "plotter#"=w351, "Plotter setup cluster.screenx"=w340, "Plotter setup cluster.screeny"=w339) -> (w357:T10)
        n185 = call <vilib>:"Add State(s) to Queue__jki_lib_state_machine.vi"("State(s) in (\"\")"=w360) -> ("States Out"=w359:string)  [unwired: 14 in]
      }
      frame "Get plotter details" {
        # "Template Separator\n(You can make a copy of, or modify, this frame)"
        n186 = Unbundle By Name(w379) -> ("plotter#"=w389:string)
        n187 = call "preset SQL Queries.vi"("error in (no error)"=w376, "Device/Devicetype name\n/Plotter.id/ScanName#"=w389, "Preset Query"=Preset_Query_Enum."Get plotter details") -> ("error out"=w375:errorcluster, "data"=w388:string[][])  [unwired: 6 in, 1 out]
        "plotter details" <- w388
        n188 = Index Array(array=w388, index (row)=1) -> (element=w386:string[])  [unwired: 1 in]
        n189 = Index Array(array=w386) -> (element #2=w385:string, element #3=w383:string, element #4=w381:string, element #5=w380:string, element #6=w374:string)  [unwired: 6 in, 1 out]
        n190 = Decimal String To Number(string=w385) -> (number=w384:i32)  [unwired: 2 in, 1 out]
        n191 = Decimal String To Number(string=w383) -> (number=w382:i32)  [unwired: 2 in, 1 out]
        n192 = Bundle By Name(cluster=T8 {"screenx"=25, "screeny"=75, "variable1"="", "variable2"="", "name"=""} ("Plotter setup cluster"), "screenx"=w384, "screeny"=w382, "variable1"=w381, "variable2"=w380, "name"=w374) -> (w377:T8)
        n193 = Bundle By Name(cluster=w379, "Plotter setup cluster"=w377) -> (w378:T10)
        n194 = call <vilib>:"Add State(s) to Queue__jki_lib_state_machine.vi"("State(s) in (\"\")"=w393) -> ("States Out"=w392:string)  [unwired: 14 in]
      }
      frame "Main: Read Expt Config" {
        # "todo. get rid of the copy of parameters"
        # "Reads the configuration for a particular experiment. eg TREX default would save spectrum mode image and\nget back centroid etc."
        n195 = Unbundle By Name(w420) -> ("Experiment name"=w402:string)
        n196 = call "preset SQL Queries.vi"("error in (no error)"=w401, "Expt name / MCIP/ Variable/Preset Name"=w402, "Preset Query"=Preset_Query_Enum."Get experiment basic properties") -> ("error out"=w400:errorcluster, "1st column 1st data"=w398:string[], "data"=w397:string[][])  [unwired: 6 in]
        n197 = Index Array(array=w398) -> (element=w404:string)  [unwired: 1 in]
        n198 = Index Array(array=w397, index (row)=1, index (col)=2 ("disabled index (col)")) -> (element=w394:string)
        n199 = call "preset SQL Queries.vi"("error in (no error)"=w400, "Expt name / MCIP/ Variable/Preset Name"=w402, "Preset Query"=Preset_Query_Enum."Get expt devices with data to get") -> ("error out"=w418:errorcluster, "data"=w415:string[][])  [unwired: 6 in, 1 out]
        n200 = Decimal String To Number(string=w394) -> (number=w399:i32)  [unwired: 2 in, 1 out]
        n201 = Delete From Array(array=w415, index (row)=0) -> (array with subset deleted=w417:string[][])  [unwired: 2 in, 1 out]
        n202 = Index Array(array=w417, index (col)=0 ("disabled index (col)")) -> (element=w410:string[])  [unwired: 1 in]
        "devices to get data from" <- w410
        n203 = call "preset SQL Queries.vi"("error in (no error)"=w418, "Expt name / MCIP/ Variable/Preset Name"=w402, "Preset Query"=Preset_Query_Enum."Get expt devices and variables (with data to get)") -> ("error out"=w411:errorcluster, "data"=w409:string[][])  [unwired: 6 in, 1 out]
        "parameters to get" <- w409
        n204 = Bundle By Name(cluster=w420, "expt config file array"=w409, "ScanData to receive"=w409, "Device Names for scan data"=w410) -> (w419:T10)
        n205 = call "Plotter FGV Cluster.vi"("Function"=enum16{"Read", "Write", "Clear"}."Read") -> ("Cluster out"=w405:T4)  [unwired: 9 in, 1 out]
        n206 = Bundle By Name(cluster=w405, "Multicast Address"=w404, "Mcast Port"=w399) -> (w403:T4)
        n207 = call <vilib>:"Add State(s) to Queue__jki_lib_state_machine.vi"("State(s) in (\"\")"=w422) -> ("States Out"=w421:string)  [unwired: 14 in]
        n208 = call "Plotter FGV Cluster.vi"("Function"=enum16{"Read", "Write", "Clear"}."Write", "Cluster in"=w403) -> ()  [unwired: 8 in, 2 out]
      }
      frame "Get List of Axis Names" {
        # "Increments scan #, resets shot number and sends list of states to execute at the start of a scan. Only does this\nif variable for scan is numeric."
        n209 = Unbundle By Name(w428) -> ("ScanData to receive"=w426:string[][])
        n210 = Delete From Array(array=w426, index (row)=0) -> (array with subset deleted=w424:string[][])  [unwired: 2 in, 1 out]
        n211 = Index Array(array=w424, index (col) #1=0 ("disabled index (col)"), index (col) #2=1 ("index (col)")) -> (element #1=w430:string[], element #2=w429:string[])  [unwired: 2 in]
        n212 = for {
          tunnel: w430 -> [w438] mode=indexing
          tunnel: w429 -> [w437] mode=indexing
          tunnel: [w436] -> w423 mode=indexing
          n213 = Concatenate Strings(w438, " " ("string"), w437) -> (w436:string)
        }
        "Axis Name List" <- w423
        n214 = Bundle By Name(cluster=w428, "Data titles from config array"=w423) -> (w427:T10)
        n215 = property on="Y Axis 2" class="Ring (strict)"("Strings []"=w423) -> ()  [unwired: 2 in, 2 out]
        n216 = property on="Y Axis" class="Ring (strict)"("Strings []"=w423) -> ()  [unwired: 2 in, 2 out]
        n217 = property on="X Axis" class="Ring (strict)"("Strings []"=w423) -> ()  [unwired: 2 in, 2 out]
        n218 = call <vilib>:"Add State(s) to Queue__jki_lib_state_machine.vi"("State(s) in (\"\")"=w435) -> ("States Out"=w434:string)  [unwired: 14 in]
      }
      frame "Get Default Y Axis" {
        # "Increments scan #, resets shot number and sends list of states to execute at the start of a scan. Only does this\nif variable for scan is numeric."
        n219 = property on="Y Axis" class="Ring (strict)"() -> ("Strings []"=w441:string[])  [unwired: 2 in, 2 out]
        n220 = property on="Y Axis 2" class="Ring (strict)"() -> ("Strings []"=w440:string[])  [unwired: 2 in, 2 out]
        n221 = case shown="True" TRUE {
          tunnel: w447 -> [_ w459]
          tunnel: ["vc" ("variable1") w456] -> w446
          tunnel: ["xcv" ("variable2") w453] -> w445
          tunnel: w441 -> [_ w455]
          tunnel: w440 -> [_ w454]
          frame False {
          }
          frame True {
            n222 = Unbundle By Name(w459) -> ("Plotter setup cluster.variable1"=w456:string, "Plotter setup cluster.variable2"=w453:string)
            "Y Axis Default name" <- w456
            "Y Axis Default name 2" <- w453
            n223 = Search 1D Array(1D array=w454, element=w453) -> (index of element=w457:i32)  [unwired: 1 in]
            n224 = Search 1D Array(1D array=w455, element=w456) -> (index of element=w458:i32)  [unwired: 1 in]
            n225 = local write "Y Axis"(w458) -> ()
            n226 = local write "Y Axis 2"(w457) -> ()
          }
        }
        n227 = stacked-sequence {
          tunnel: w446 -> [w463 w467]
          tunnel: w445 -> [w462 w466]
          tunnel: 0 ("Active Y Scale") -> [w461 w465]
          tunnel: 1 ("Active Y Scale") -> [w460 w464]
          frame #0 {
            n228 = property on="xy graph" class="XYGraph (strict)"("ActYScl"=w461, "YScale.NameLbl.Text"=w463, "ActYScl"=w460, "YScale.NameLbl.Text"=w462) -> ()  [unwired: 2 in, 2 out]
          }
          frame #1 {
            n229 = property on="xy graph bin" class="XYGraph (strict)"("ActYScl"=w465, "YScale.NameLbl.Text"=w467, "ActYScl"=w464, "YScale.NameLbl.Text"=w466) -> ()  [unwired: 2 in, 2 out]
          }
        }
        n230 = call <vilib>:"Add State(s) to Queue__jki_lib_state_machine.vi"("State(s) in (\"\")"=w450) -> ("States Out"=w449:string)  [unwired: 14 in]
      }
      frame "Main: Set Panel Postion" {
        # "Reads the configuration for a particular experiment. eg TREX default would save spectrum mode image and\nget back centroid etc."
        n231 = disable-structure shown="Enabled" {
          disable-tunnel: w470 -> [w478 _]
          disable-tunnel: w469 -> [w474 w506]
          disable-tunnel: [w473 w506] -> w468
          frame Enabled {
            n232 = Unbundle By Name(w478) -> ("Plotter setup cluster.screenx"=w476:i16, "Plotter setup cluster.screeny"=w475:i16)
            n233 = control-ref of="This VI"() -> (w477:refnum<vi>)
            n234 = disable-structure shown="Enabled" {
              disable-tunnel: w477 -> [w485 w505]
              disable-tunnel: w476 -> [w484 w496]
              disable-tunnel: w475 -> [w483 w493]
              disable-tunnel: w474 -> [w480 _]
              disable-tunnel: [w479 _] -> w473
              frame Disabled {
                n235 = property on="Tab Control" class="TabCtl (strict)"() -> ("PaneWidth"=w491:u32, "PaneHeight"=w490:u32)  [unwired: 2 in, 2 out]
                n236 = Add(x=w490, y=u32 25) -> (x+y=w481:u32)
                n237 = Add(x=u32 15, y=w491) -> (x+y=w482:u32)
                n238 = Bundle By Name(cluster="Cluster", "Left"=w484, "Top"=w483, "Width"=w482, "Height"=w481) -> (w486:T2)
                n239 = call "set panel position MC only.vi"("error out 2"=w480, "Cluster"=w486, "This VI"=w485) -> ("error out"=w479:errorcluster)
              }
              frame Enabled {
                n240 = property class="VI"(reference=w505) -> (reference out=w504:refnum<vi>, "Front Panel.WinBounds"=w499:T11)  [unwired: 1 in, 1 out]
                n241 = Unbundle By Name(w499) -> ("Left"=w500:i16, "Top"=w502:i16, "Right"=w501:i16, "Bottom"=w503:i16)
                n242 = Subtract(x=w503, y=w502) -> (x-y=w494:i16)
                n243 = Subtract(x=w501, y=w500) -> (x-y=w497:i16)
                n244 = Add(x=w493, y=w494) -> (x+y=w492:i16)
                n245 = Add(x=w496, y=w497) -> (x+y=w495:i16)
                n246 = Bundle By Name(cluster=w499, "Left"=w496, "Top"=w493, "Right"=w495, "Bottom"=w492) -> (w498:T11)
                n247 = property class="VI"(reference=w504, "Front Panel.WinBounds"=w498) -> ()  [unwired: 1 in, 2 out]
              }
            }
          }
          frame Disabled {
          }
        }
        n248 = call <vilib>:"Add State(s) to Queue__jki_lib_state_machine.vi"("State(s) in (\"\")"=w472) -> ("States Out"=w471:string)  [unwired: 14 in]
      }
      frame "Main: Get Device Configs" {
        # "Reads the configuration for a particular experiment. eg TREX default would save spectrum mode image and\nget back centroid etc."
        n249 = call "preset SQL Queries.vi"("error in (no error)"=w508, "Preset Query"=Preset_Query_Enum."Get all devices basic properties") -> ("error out"=w507:errorcluster, "data"=w509:string[][])  [unwired: 7 in, 1 out]
        "All Devices Core Info" <- w509
        n250 = Bundle By Name(cluster=w511, "All Devices Core Info"=w509) -> (w512:T10)
        n251 = call <vilib>:"Add State(s) to Queue__jki_lib_state_machine.vi"("State(s) in (\"\")"=w514) -> ("States Out"=w513:string)  [unwired: 14 in]
      }
      frame "Plot" {
        # "Your code here.\n(You can make a copy of, or modify, this frame)"
        n252 = Unbundle By Name(w539) -> ("TDMS file path"=w537:path)
        "TDMS file path" <- w537
        n253 = call "Plotter FGV Cluster.vi"("error in"=w522, "Function"=enum16{"Read", "Write", "Clear"}."Read") -> ("error out"=w529:errorcluster, "Cluster out"=w531:T4)  [unwired: 8 in]
        n254 = Bundle By Name(cluster=w531, "Plotter Busy"=TRUE) -> (w528:T4)
        n255 = Select(t="file path", s="FilePath", f=w537) -> (s? t:f=w516:path)
        "Path used" <- w516
        n256 = call-poly <userlib>:"Convert File Extension__ogtk.vi"("file name"=w516) -> ("new filename"=w515:path)  [unwired: 1 in, 1 out]
        n257 = call "Plotter FGV Cluster.vi"("error in"=w529, "Function"=enum16{"Read", "Write", "Clear"}."Write", "Cluster in"=w528) -> ("error out"=w533:errorcluster, "Cluster out"=w525:T4)  [unwired: 7 in]
        n258 = Strip Path(path=w515) -> (name=→"Scan":string)  [unwired: 1 out]
        n259 = Bundle By Name(cluster=w525, "Plotter Busy"=FALSE) -> (w524:T4)
        n260 = call <vilib>:"Check if File or Folder Exists.vi"("error in (no error)"=w533, "path"=w516) -> ("error out"=w534:errorcluster, "file or folder exists?"=w536:bool, "dup path"=w535:path)  [unwired: 7 in]
        n261 = case shown="True" w536 {
          tunnel: w535 -> [_ w545]
          tunnel: w539 -> [_ w548]
          tunnel: w534 -> [w542 w544]
          tunnel: w520 -> [_ w547]
          tunnel: "FilePath" -> [_ w546]
          tunnel: [w542 w543] -> w518
          frame False {
          }
          frame True {
            n262 = stacked-sequence {
              seq-local: [w561 _ _ _ _] -> [_ _ _ w619 w629]
              seq-local: [_ _ _ w618 _] -> [_ _ _ _ _]
              tunnel: w545 -> [w558 _ _ w621 w635]
              tunnel: w548 -> [_ w591 _ _ w634]
              tunnel: w547 -> [_ _ _ _ w636]
              tunnel: w546 -> [w551 _ w597 _ _]
              tunnel: w544 -> [w562 _ _ _ _]
              tunnel: [_ _ _ _ w628] -> w543
              frame #0 {
                n263 = disable-structure shown="Disabled" {
                  disable-tunnel: w558 -> [w575 _]
                  disable-tunnel: [w572 FALSE] -> w557
                  frame Disabled {
                    n264 = Get File Size(file=w575) -> (size (in bytes)=w574:i64)  [unwired: 1 in, 2 out]
                    n265 = feedback #1(i64 0 ("size (in bytes)")) -> (w573:i64)
                    n266 = feedback-in #1(w574) -> ()
                    n267 = Equal?(x=w574, y=w573) -> (x = y?=w572:bool)
                  }
                  frame Enabled {
                  }
                }
                n268 = case shown="False" w557 {
                  tunnel: w562 -> [w581 w582]
                  tunnel: [w580 w582] -> w561
                  tunnel: [w579 w583] -> w552
                  tunnel: w558 -> [w578 _]
                  tunnel: w551 -> [w577 _]
                  frame False {
                    n269 = call "Read TDMS - LOASIS scan data.vi"("error in (no error)"=w581, "UsingFilePath"=w577, "file path"=w578) -> ("error out"=w580:errorcluster, "device data Spreadsheet format"=w579:string[][])  [unwired: 6 in, 1 out]
                  }
                  frame True {
                    n270 = local read "data"() -> (w583:string[][])
                  }
                }
                n271 = local read "data"() -> (w549:string[][])
                n272 = Index Array(array=w552, index (row)=1, index (col)=0) -> (element=w553:string)
                n273 = case shown="Default" w553 {
                  tunnel: w552 -> [w567 w570]
                  tunnel: [w563 w569] -> w550
                  tunnel: w549 -> [w564 _]
                  frame Default {
                    n274 = Index Array(array=w567, index (row)=1) -> (element=w565:string[])  [unwired: 1 in]
                    n275 = Build Array (concatenate)(w564, w565) -> (w563:string[][])
                  }
                  frame "1", "2" {
                    n276 = Build Array (concatenate)(string[][] [] ("device names"), w570) -> (w569:string[][])
                  }
                }
                "data" <- w550
                n277 = call "replace variable names with aliases.vi"("device data Spreadsheet format in"=w550) -> ("device data spreadsheet with alias"=→"tdms data":string[][])  [unwired: 2 in]
                n278 = Index Array(array=w550, index (row)=0) -> (element=w559:string[])  [unwired: 1 in]
                n279 = property on="Y Axis 2" class="Ring (strict)"("Strings []"=w559) -> ()  [unwired: 2 in, 2 out]
                n280 = property on="X Axis" class="Ring (strict)"("Strings []"=w559) -> ()  [unwired: 2 in, 2 out]
                n281 = property on="Y Axis" class="Ring (strict)"("Strings []"=w559) -> ()  [unwired: 2 in, 2 out]
              }
              frame #1 {
                n282 = case shown="True" "override" {
                  tunnel: w591 -> [w594 _]
                  tunnel: [w593 "y axis override"] -> w589
                  tunnel: [w592 "y axis 2 override"] -> w586
                  frame False {
                    n283 = Unbundle By Name(w594) -> ("Plotter setup cluster.variable1"=w593:string, "Plotter setup cluster.variable2"=w592:string)
                  }
                  frame True {
                  }
                }
                n284 = property on="Y Axis 2" class="Ring (strict)"() -> ("Strings []"=w587:string[])  [unwired: 2 in, 2 out]
                n285 = property on="Y Axis" class="Ring (strict)"() -> ("Strings []"=w590:string[])  [unwired: 2 in, 2 out]
                n286 = Search 1D Array(1D array=w587, element=w586) -> (index of element=w585:i32)  [unwired: 1 in]
                n287 = Search 1D Array(1D array=w590, element=w589) -> (index of element=w588:i32)  [unwired: 1 in]
                n288 = local write "Y Axis 2"(w585) -> ()
                n289 = local write "Y Axis"(w588) -> ()
              }
              frame #2 {
                n290 = case shown="False" w597 {
                  frame False {
                    n291 = case shown="True" "Override" {
                      tunnel: [w605 "x axis override"] -> w604
                      frame False {
                        n292 = local read "x axis name"() -> (w605:string)
                      }
                      frame True {
                      }
                    }
                    n293 = property on="X Axis" class="Ring (strict)"() -> ("Strings []"=w600:string[])  [unwired: 2 in, 2 out]
                    n294 = Search 1D Array(1D array=w600, element=w604) -> (index of element=w601:i32)  [unwired: 1 in]
                    n295 = Less Than 0?(x=w601) -> (x < 0?=w603:bool)
                    n296 = case shown="True" w603 {
                      tunnel: [w607 w610] -> w602
                      tunnel: w601 -> [w607 _]
                      tunnel: w600 -> [_ w609]
                      tunnel: "Rep Rate shot #" ("element") -> [_ w608]
                      frame False {
                      }
                      frame True {
                        n297 = Search 1D Array(1D array=w609, element=w608) -> (index of element=w610:i32)  [unwired: 1 in]
                      }
                    }
                    n298 = local write "X Axis"(w602) -> ()
                  }
                  frame True {
                  }
                }
              }
              frame #3 {
                n299 = disable-structure shown="Enabled" {
                  disable-tunnel: w621 -> [w625 _]
                  disable-tunnel: w619 -> [w624 w626]
                  disable-tunnel: [w623 w626] -> w618
                  disable-tunnel: [w622 w627] -> w611
                  frame Disabled {
                    n300 = call "Read TDMS - LOASIS scan data.vi"("error in (no error)"=w624, "file path"=w625) -> ("error out"=w623:errorcluster, "device data Spreadsheet format"=w622:string[][])  [unwired: 7 in, 1 out]
                  }
                  frame Enabled {
                    n301 = local read "tdms data"() -> (w627:string[][])
                  }
                }
                n302 = control-ref of="Y Axis 2"() -> (w616:refnum<vi>)
                n303 = control-ref of="xy graph"() -> (w617:refnum<vi>)
                n304 = control-ref of="X Axis"() -> (w614:refnum<vi>)
                n305 = control-ref of="Y Axis"() -> (w615:refnum<vi>)
                n306 = Bundle By Name(cluster=T9 {"Ring Refnum x"=refnum, "Ring Refnum y"=refnum, "Ring Refnum y 2"=refnum, "XY Graph Refnum"=refnum} ("Cluster"), "Ring Refnum x"=w614, "Ring Refnum y"=w615, "Ring Refnum y 2"=w616, "XY Graph Refnum"=w617) -> (w612:T9)
                n307 = call "Select axes.vi"("Cluster"=w612, "output array"=w611) -> ("XY Graph"=→"xy graph":cluster{dbl[], dbl[]}[])  [unwired: 4 in, 2 out]
              }
              frame #4 {
                n308 = local read "x axis name"() -> (w631:string)
                n309 = Unbundle By Name(w634) -> ("Plotter setup cluster.variable1"=w632:string, "Plotter setup cluster.variable2"=w633:string, "Plotter setup cluster.name"=w630:string)
                n310 = case shown="\"nobin\", Default" w636 {
                  tunnel: w635 -> [_ w652]
                  tunnel: w633 -> [_ w644]
                  tunnel: w632 -> [_ w646]
                  tunnel: w631 -> [_ w643]
                  tunnel: w630 -> [_ w651]
                  tunnel: w629 -> [w637 w639]
                  tunnel: [w637 w638] -> w628
                  frame "nobin", Default {
                  }
                  frame "bin" {
                    n311 = call "Read TDMS - LOASIS scan data.vi"("error in (no error)"=w639, "file path"=w652) -> ("error out"=w653:errorcluster, "device data Spreadsheet format"=w645:string[][])  [unwired: 7 in, 1 out]
                    "device data Spreadsheet format" <- w645
                    n312 = call "binbyStepIndex02.vi"("y1 col name"=w646, "x col name"=w643, "device data Spreadsheet format"=w645) -> ("XY Graph 2"=w642:cluster{"ind":dbl[], "ini2":dbl[]}[])  [unwired: 6 in, 2 out]
                    n313 = call "binbyStepIndex02.vi"("y1 col name"=w644, "x col name"=w643, "device data Spreadsheet format"=w645) -> ("XY Graph 2"=w641:cluster{"ind":dbl[], "ini2":dbl[]}[])  [unwired: 6 in, 2 out]
                    n314 = Build Array (concatenate)(w642, w641) -> (→"xy graph bin":cluster{"ind":dbl[], "ini2":dbl[]}[])
                    n315 = call "tdms path to plotter png path.vi"("error in"=w653, "plotter name"=w651, "TDMS Path"=w652) -> ("error out"=w638:errorcluster, "binned plotter png save path"=w648:path, "plotter png save path"=w647:path)  [unwired: 6 in]
                    n316 = control-ref of="xy graph bin"() -> (w650:refnum<vi>)
                    n317 = control-ref of="xy graph"() -> (w649:refnum<vi>)
                    n318 = call "plotter save png.vi"("binned plotter png save path"=w648, "plotter png save path"=w647, "XYGraph Refnum in"=w650, "XYGraph in"=w649) -> ()  [unwired: 8 in]
                  }
                }
              }
            }
          }
        }
        n319 = call <vilib>:"Add State(s) to Queue__jki_lib_state_machine.vi"("State(s) in (\"\")"=w541) -> ("States Out"=w540:string)  [unwired: 14 in]
        n320 = call "Plotter FGV Cluster.vi"("error in"=w518, "Function"=enum16{"Read", "Write", "Clear"}."Write", "Cluster in"=w524) -> ("error out"=w521:errorcluster)  [unwired: 7 in, 1 out]
      }
      frame "19" {
        # "Your code here.\n(You can make a copy of, or modify, this frame)"
        n321 = call <vilib>:"Add State(s) to Queue__jki_lib_state_machine.vi"("State(s) in (\"\")"=w657) -> ("States Out"=w656:string)  [unwired: 14 in]
      }
      frame "get panel position" {
        # "Your code here.\n(You can make a copy of, or modify, this frame)"
        n322 = control-ref of="This VI"() -> (w664:refnum<vi>)
        n323 = call "get vi screen position.vi"("error in"=w663, "This VI"=w664) -> ("error out"=w662:errorcluster, "Front Panel Window:Panel Bounds"=w661:T11)  [unwired: 8 in]
        n324 = Unbundle By Name(w661) -> ("Left"=w660:i16, "Top"=w659:i16)
        n325 = Bundle("Left"=w660, "Top"=w659) -> (→"Screen\nPosition":cluster{"Left":i16, "Top":i16})  [unwired: 1 in]
        n326 = call <vilib>:"Add State(s) to Queue__jki_lib_state_machine.vi"("State(s) in (\"\")"=w667) -> ("States Out"=w666:string)  [unwired: 14 in]
      }
    }
    "error out 2" <- w88
  }
  n327 = disable-structure shown="Disabled" {
    frame Disabled {
      n328 = call "binning for loasis TDMS plotter.vi"() -> ()  [unwired: 11 in, 1 out]
    }
    frame Enabled {
    }
  }
